vi "writeToXML.vi"(8 "error in (no error)":errorcluster, 10 "classLabel":string, 11 "Target in":refnum<class "Target.lvclass">) -> (0 "error out":errorcluster, 2 "XML out":string, 3 "Target out":refnum<class "Target.lvclass">)   [LabVIEW 2014, in "TCSDataDefinitions.lvlib" / "TCSCommand.lvlib" / "TargetConfiguration.lvlib" / "Target.lvlib" / "Target.lvclass"]
uses:
  Target/Target.lvclass
  Target/Target.lvclass/Target.ctl
  Difftrack/Difftrack.lvclass
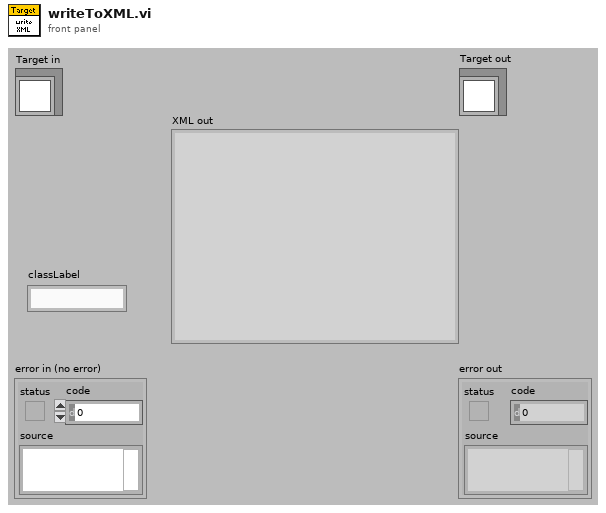
[diagram p1: front panel]
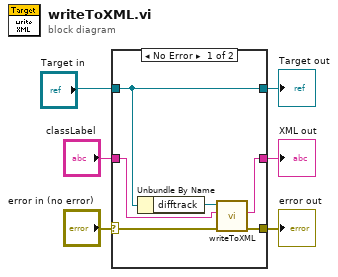
[diagram p0: block diagram]
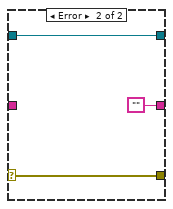
[diagram p2: hidden frame]
diagram:
  n1 = case shown="No Error" "error in (no error)" {
    selector: "error in (no error)" -> [w11 w15]
    tunnel: [w9 w15] -> w5
    tunnel: [w12 w14] -> w4
    tunnel: "Target in" -> [w12 w14]
    tunnel: "classLabel" -> [w10 _]
    tunnel: [w8 ""] -> w2
    frame No Error {
      n2 = Unbundle By Name(w12) -> ("difftrack"=w7:refnum<class "Difftrack.lvclass">)
      n3 = call-dynamic "writeToXML.vi"("error in (no error)"=w11, "ClassLabel"=w10, "Difftrack in"=w7) -> ("error out"=w9:errorcluster, "XML out"=w8:string)  [unwired: 6 in, 1 out]
    }
    frame Error {
    }
  }
  "error out" <- w5
  "Target out" <- w4
  "XML out" <- w2
